vi "Get ROI and Metadata.vi"(8 "Offset Bytes":i32, 9 "Metadata Bytes":i32, 10 "ROI Bytes":i32, 11 "Bytes":u8[](array[numeric])) -> (2 "Metadata":u8[](array[numeric]), 3 "ROI data":u8[](array[numeric]))   [LabVIEW 2019, in "Picam.lvclass"]
uses:
  Picam.lvclass
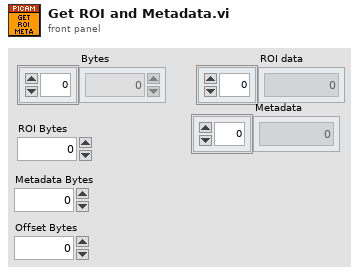
[diagram p1: front panel]
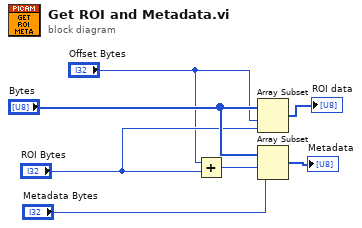
[diagram p0: block diagram]
diagram:
  n1 = Add(x="Offset Bytes", y="ROI Bytes") -> (x+y=w2:i32)
  n2 = Array Subset(array="Bytes", index="Offset Bytes", length="ROI Bytes") -> (→"ROI data":u8[])
  n3 = Array Subset(array="Bytes", index=w2, length="Metadata Bytes") -> (→"Metadata":u8[])
